vi "SAVE LOOP TIMES.vi"(0 "time this loop":dbl, 5 "time last loop":dbl, 9 "System loop time stack":string, 11 "LOOP NAME":string, 12 "loop iteration":i32, 13 "milliseconds to wait":u32) -> (15 "error out":errorcluster)   [LabVIEW 2017]
uses:
  <vilib>/Rock Robotics/Network Tables/NT Read Number.vi
  <vilib>/Rock Robotics/Network Tables/NT Write Boolean.vi
  <vilib>/Rock Robotics/Network Tables/NT Write Number.vi
panel:
  out "loop slow?":bool
  out "elapsed time":dbl
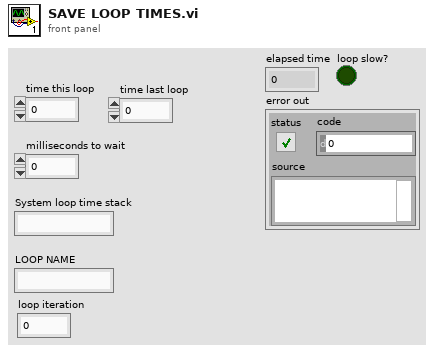
[diagram p1: front panel]
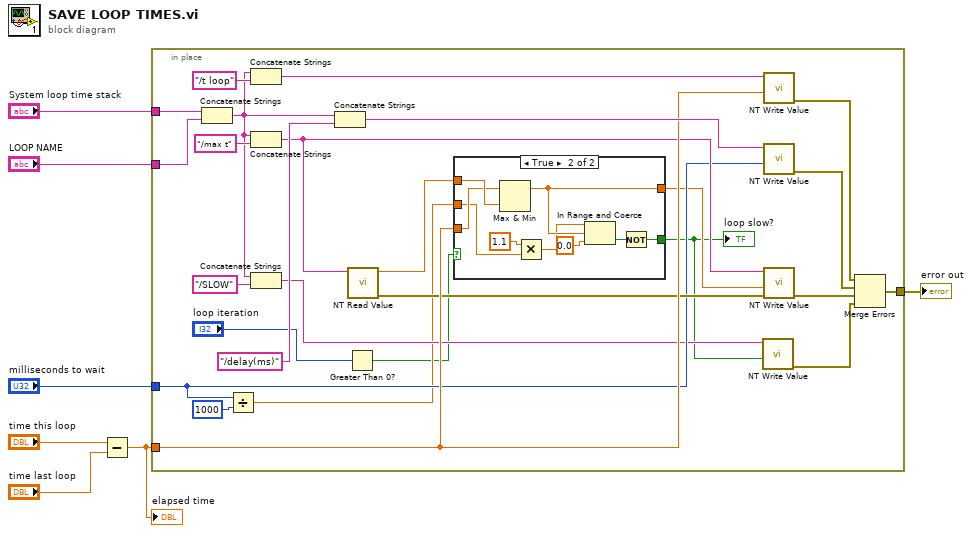
[diagram p0: block diagram]
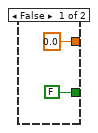
[diagram p2: hidden frame]
diagram:
  n1 = Subtract(x="time this loop", y="time last loop") -> (x-y=w5:dbl)
  "elapsed time" <- w5
  n2 = in-place {
    in-place-border: "LOOP NAME" -> [w33]
    in-place-border: "System loop time stack" -> [w19]
    in-place-border: w5 -> [w26]
    in-place-border: "milliseconds to wait" -> [w18]
    in-place-border: [w20] -> w3
    n3 = Concatenate Strings(w19, w33) -> (w15:string)
    n4 = Divide(x=w18, y=u32 1000) -> (x/y=w11:dbl)
    n5 = Concatenate Strings(w15, "/t loop" ("string")) -> (w32:string)
    n6 = Concatenate Strings(w15, "/max t" ("string")) -> (w25:string)
    n7 = Concatenate Strings(w15, "/SLOW" ("string")) -> (w14:string)
    n8 = Concatenate Strings(w15, "/delay(ms)" ("string")) -> (w30:string)
    n9 = Greater Than 0?(x="loop iteration") -> (x > 0?=w8:bool)
    n10 = call-poly <vilib>:"NT Read Value.vi"("Name"=w25) -> ("error out"=w23:errorcluster, "Numeric"=w27:dbl)  [unwired: 9 in]
    n11 = case shown="True" w8 {
      tunnel: w27 -> [_ w44]
      tunnel: w26 -> [_ w43]
      tunnel: [0.0 w41] -> w12
      tunnel: w11 -> [_ w38]
      tunnel: [FALSE w37] -> w10
      frame False {
      }
      frame True {
        n12 = Max & Min(x=w43, y=w44) -> (max(x,y)=w41:dbl)  [unwired: 1 out]
        n13 = Multiply(x=1.1, y=w38) -> (x*y=w40:dbl)
        n14 = In Range and Coerce(upper limit=w40, x=w41, lower limit=0.0) -> (In Range?=w42:bool)  [unwired: 1 out]
        n15 = Not(x=w42) -> (.not. x?=w37:bool)
      }
    }
    "loop slow?" <- w10
    n16 = call-poly <vilib>:"NT Write Value.vi"("Boolean"=w10, "Name"=w14) -> ("error out"=w16:errorcluster)  [unwired: 9 in]
    n17 = call-poly <vilib>:"NT Write Value.vi"("Numeric"=w26, "Name"=w32) -> ("error out"=w22:errorcluster)  [unwired: 9 in]
    n18 = call-poly <vilib>:"NT Write Value.vi"("Numeric"=w18, "Name"=w30) -> ("error out"=w21:errorcluster)  [unwired: 9 in]
    n19 = call-poly <vilib>:"NT Write Value.vi"("error in"=w23, "Numeric"=w12, "Name"=w25) -> ("error out"=w24:errorcluster)  [unwired: 8 in]
    n20 = Merge Errors(w22, w21, w24, w16) -> (w20:errorcluster)
  }
  "error out" <- w3
